vi "Start.vi"(6 "timeout (ms)":i32=5000, 8 "error in":errorcluster, 10 "FTE (ns)":u64, 11 "gRPC ID":T1) -> (0 "error out":errorcluster, 3 "gRPC ID out":T1)   [LabVIEW 2021, in "CoreGrpcClientWrapper.lvlib"]
uses:
  <vilib>/gRPC/LabVIEW gRPC Library/Shared/grpcId.ctl
  CIF_Plugin_Core_client/RPC Messages/cif_plugincore_FutureTimeEvent.ctl
  CoreGrpcClientWrapper.lvlib
  CIF_Plugin_Core_client/CIF_Plugin_Core_client.lvlib
  <vilib>/gRPC/LabVIEW gRPC Library/grpc-lvsupport-release.lvlib
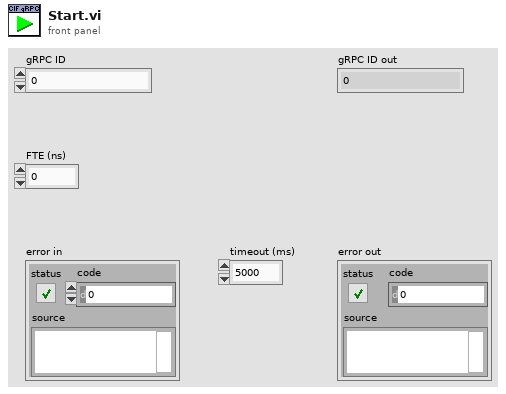
[diagram p1: front panel]
types:
  T1 = typedef "grpc-lvsupport-release.lvlib/grpcId.ctl" = u64
  T2 = typedef "CIF_Plugin_Core_client.lvlib/cif_plugincore_FutureTimeEvent.ctl" = cluster{"fte_ns":u64}
  T3 = typedef "CIF_Plugin_Core_client.lvlib/cif_plugincore_Status.ctl" = cluster{"code":i32, "message":string}
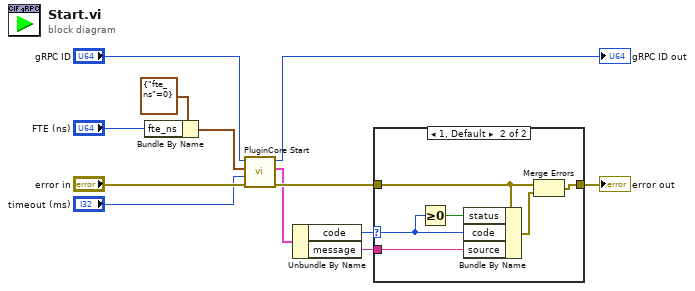
[diagram p0: block diagram]
diagram:
  n1 = Bundle By Name(cluster=T2 {"fte_ns"=0} ("Request Data"), "fte_ns"="FTE (ns)") -> (w6:T2)
  n2 = call "PluginCore Start.vi"("error in"="error in", "timeout (ms)"="timeout (ms)", "Request Data"=w6, "gRPC ID"="gRPC ID") -> ("error out"=w4:errorcluster, "Response Data"=w1:T3, "gRPC ID out"=→"gRPC ID out":T1)  [unwired: 5 in]
  n3 = Unbundle By Name(w1) -> ("code"=w2:i32, "message"=w5:string)
  n4 = case shown="1, Default" w2 {
    selector: w2 -> [_ w14]
    tunnel: w5 -> [_ w18]
    tunnel: w4 -> [w13 w17]
    tunnel: [w13 w15] -> w3
    frame 0 {
    }
    frame 1, Default {
      n5 = Greater Or Equal To 0?(x=w14) -> (x >= 0?=w19:bool)
      n6 = Bundle By Name(cluster=w17, "status"=w19, "code"=w14, "source"=w18) -> (w16:errorcluster)
      n7 = Merge Errors(w17, w16) -> (w15:errorcluster)
    }
  }
  "error out" <- w3
